vi "Serial port communication logger.vi"() -> ()   [LabVIEW 2016]
doc: "This example performs a serial port write and a serial port read. The parameters set for the serial port must match the parameters of the connected instrument or device. The VISA Configure Serial Port VI sets the configuration parameters. The front panel displays the controls used to configure the basic parameters, such as baud rate, data bits, and parity. The VI passes the VISA resource name to other VIs that perform operations on that VISA resource. The VISA Write function sends a command to the serial device and the VISA Read function returns data based on the command. The VISA Close function then closes the reference to the serial device. It is important to close the reference; otherwise, further communication through that port might not be possible."
uses:
  C:/Program Files/National Instruments/LabVIEW 2015/examples/Instrument IO/Serial/support/Serial - Settings.ctl
  <vilib>/Instr/_visa.llb/VISA Configure Serial Port (Instr).vi
panel:
  out "T reading":dbl format="%.3g"
  in  "Sampling rate (ms)":u32
  in  "stop":bool
  in  "Command (RT, RS..)":string(combo)="RT"
  out "Response":string
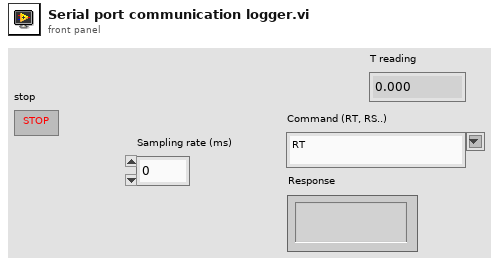
[diagram p1: front panel]
types:
  T1 = typedef "Serial - Settings.ctl" = cluster{"baud rate":u32, "data bits":u16, "parity":enum16{"None", "Odd", "Even", "Mark", "Space"}, "stop bits":u16, "flow control":u16}
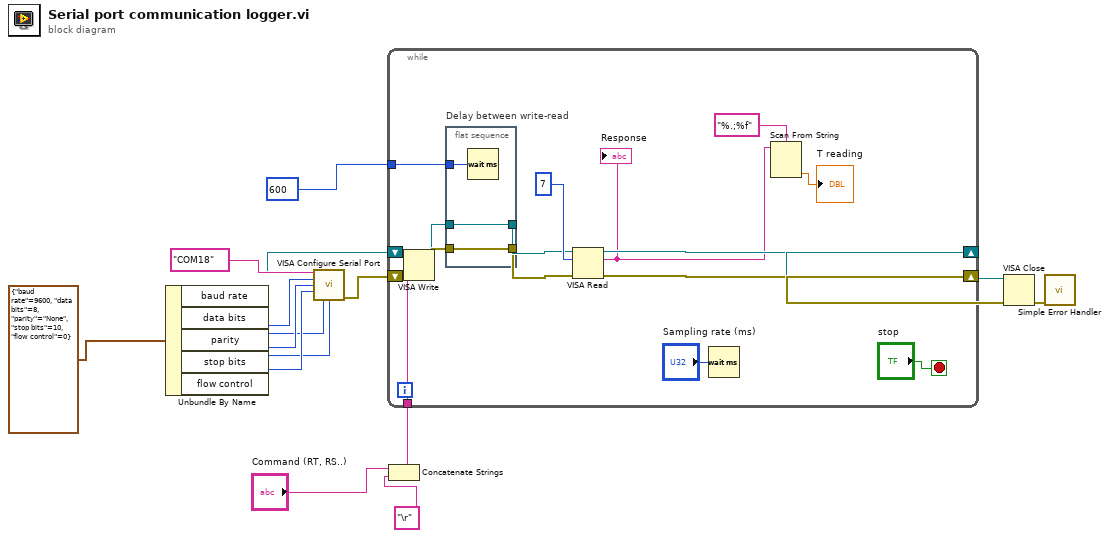
[diagram p0: block diagram]
diagram:
  n1 = Unbundle By Name(T1 {"baud rate"=9600, "data bits"=8, "parity"=enum."None", "stop bits"=10, "flow control"=0} ("Serial Settings")) -> ("baud rate"=w8:u32, "data bits"=w7:u16, "parity"=w6:enum16{"None", "Odd", "Even", "Mark", "Space"}, "stop bits"=w5:u16, "flow control"=w4:u16)
  n2 = call-poly "VISA Configure Serial Port"("VISA resource name"="COM18", "baud rate (9600)"=w8, "data bits (8)"=w7, "parity (0:none)"=w6, "stop bits (10: 1 bit)"=w5, "flow control (0:none)"=w4) -> ("VISA resource name out"=w14:refnum<visa-resource-name>, "error out"=w15:errorcluster)  [unwired: 3 in, 5 out]
  n3 = Concatenate Strings("Command (RT, RS..)", "\r" ("Command (RT\\r, RS\\r)")) -> (w1:string)
  n4 = while {
    tunnel: u32 600 ("delay before read (ms)") -> [w26]
    tunnel: w1 -> [w24]
    shift-right: [w30] -> w13
    shift-left: w15 -> [w32]
    shift-right: [w29] -> w12
    shift-left: w14 -> [w31]
    stop <- "stop" stop-if-true
    n5 = VISA Write(VISA resource name=w31, write buffer=w24, error in (no error)=w32) -> (VISA resource name out=w27:refnum<visa-resource-name>, error out=w28:errorcluster)  [unwired: 1 out]
    n6 = flat-sequence "Delay between write-read" {
      tunnel: w28 -> [w34]
      tunnel: [w34] -> w21
      tunnel: w27 -> [w33]
      tunnel: [w33] -> w22
      tunnel: w26 -> [w35]
      frame #0 {
        n7 = Wait (ms)(milliseconds to wait=w35) -> ()  [unwired: 1 out]
      }
    }
    n8 = VISA Read(VISA resource name=w22, byte count=u32 7 ("bytes read"), error in (no error)=w21) -> (VISA resource name out=w29:refnum<visa-resource-name>, read buffer=w17:string, error out=w30:errorcluster)  [unwired: 1 out]
    "Response" <- w17
    n9 = Wait (ms)(milliseconds to wait="Sampling rate (ms)") -> ()  [unwired: 1 out]
    n10 = Scan From String(format string="%.;%f" ("format"), input string=w17) -> (output 1=→"T reading":dbl)  [unwired: 3 in, 3 out]
  }
  n11 = VISA Close(VISA resource name=w12, error in (no error)=w13) -> (error out=w11:errorcluster)
  n12 = call <vilib>:"Simple Error Handler.vi"("error in (no error)"=w11) -> ()  [unwired: 1 in, 8 out]
